vi "随机秘钥.vi"() -> (3 "私钥":string)   [LabVIEW 2020]
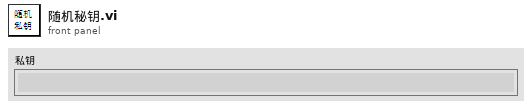
[diagram p1: front panel]
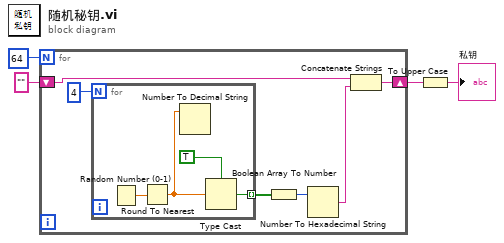
[diagram p0: block diagram]
diagram:
  n1 = for {
    N: 64 -> [_]
    shift-right: [w5] -> w2
    shift-left: "" -> [w7]
    n2 = for {
      N: 4 -> [_]
      tunnel: [w11] -> w9 mode=indexing
      n3 = Random Number (0-1)() -> (number: 0 to 1=w14:dbl)
      n4 = Round To Nearest(number=w14) -> (nearest integer value=w13:dbl)
      n5 = Number To Decimal String(number=w13) -> ()  [unwired: 1 in, 1 out]
      n6 = Type Cast(type=TRUE, x=w13) -> (*(type *) &x=w11:bool)
    }
    n7 = Boolean Array To Number(Boolean array=w9) -> (number=w8:u32)
    n8 = Number To Hexadecimal String(2:w8) -> (0:w6:string)  [unwired: 1 in]
    n9 = Concatenate Strings(w7, w6) -> (w5:string)
  }
  n10 = To Upper Case(1:w2) -> (0:→"私钥":string)
